vi "PH_AxisGUI_6P.ProcCases.vi"(0 "i ref in":refnum<vi>, 1 "selector":string, 2 "data":i8[](array[numeric]), 3 "call cluster":T1={"Object"="", "Selector"="", "CallType"=enum."synchronous", "Async Object"="", "Async Selector"="", "Data Descriptor"="", "Data"=[], "Error #"=0, "Expire"=0}, 5 "error in":errorcluster) -> (14 "i ref out":refnum<vi>, 17 "answer cluster":T1={"Object"="", "Selector"="", "CallType"=enum."synchronous", "Async Object"="", "Async Selector"="", "Data Descriptor"="", "Data"=[], "Error #"=0, "Expire"=0}, 19 "error out":errorcluster)   [LabVIEW 2014, in "PH_AxisGUI_6P.lvlib"]
doc: "This method is called by a process from within the default case in the event loop. The methods of a class that are linked to events will be called from THIS method. Add your code here."
uses:
  PH_AxisGUI_6P.lvlib
  CSCore/CSSystem/CoreDefs/CoreDefs.call_type.ctl
  CSCore/BaseProcess/BaseProcess.descriptor string definition.ctl
  CSCore/CSSystem/CoreDefs/CoreDefs.rawDataType.ctl
  PH_AxisGUI_BaseClass/PH_AxisGUI_BaseClass.lvlib
  CSCore/BaseProcess/BaseProcess.lvlib
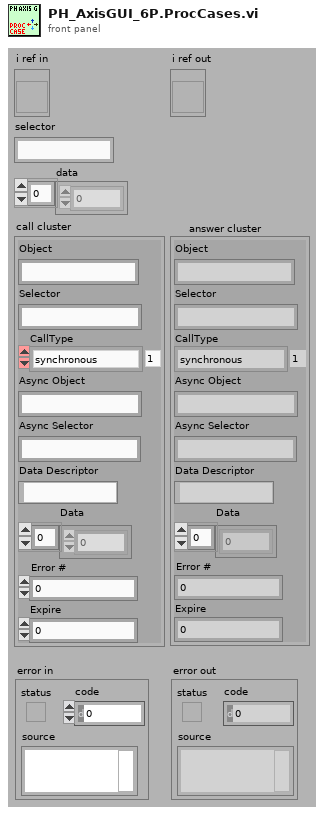
[diagram p1: front panel]
types:
  T1 = typedef "CoreDefs.call_type.ctl" = cluster{"Object":string, "Selector":string, "CallType":enum16{"simple", "synchronous", "asynchronous"}, "Async Object":string, "Async Selector":string, "Data Descriptor":T2, "Data":T3, "Error #":i32, "Expire":u32}
  T2 = typedef "BaseProcess.lvlib/BaseProcess.descriptor string definition.ctl" = string
  T3 = typedef "CoreDefs.rawDataType.ctl" = i8[]
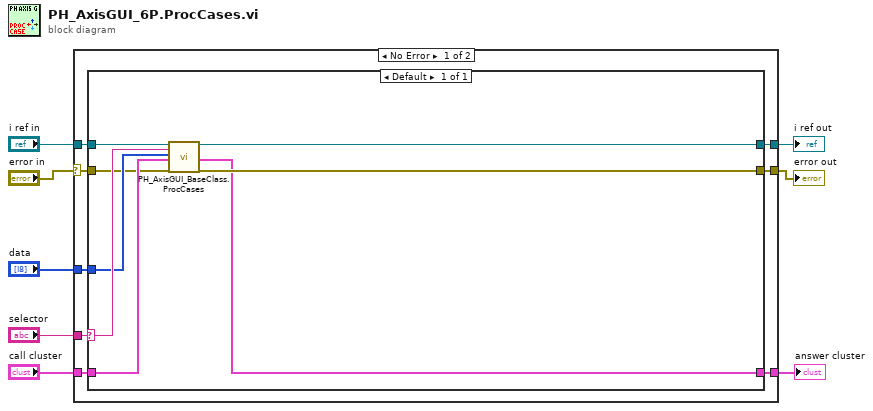
[diagram p0: block diagram]
diagram:
  n1 = case shown="No Error" "error in" {
    selector: "error in" -> [w9 w26]
    tunnel: "selector" -> [w16 _]
    tunnel: [w15 w25] -> w7
    tunnel: "call cluster" -> [w14 w25]
    tunnel: "i ref in" -> [w13 w27]
    tunnel: [w12 w27] -> w4
    tunnel: [w11 w26] -> w3
    tunnel: "data" -> [w10 _]
    frame No Error {
      n2 = case shown="Default" w16 {
        selector: w16 -> [w20]
        tunnel: w13 -> [w19]
        tunnel: [w24] -> w12
        tunnel: w14 -> [w21]
        tunnel: [w22] -> w15
        tunnel: w9 -> [w17]
        tunnel: [w23] -> w11
        tunnel: w10 -> [w18]
        frame Default {
          n3 = call "PH_AxisGUI_BaseClass.ProcCases.vi"("i ref in"=w19, "selector"=w20, "data"=w18, "call cluster"=w21, "error in"=w17) -> ("i ref out"=w24:refnum<vi>, "answer cluster"=w22:T1, "error out"=w23:errorcluster)  [unwired: 12 in]
        }
      }
    }
    frame Error {
    }
  }
  "answer cluster" <- w7
  "i ref out" <- w4
  "error out" <- w3
